vi "libdaq_adc_read_analog.vi"(0 "error in (no error)":errorcluster, 1 "device_name":string, 2 "module_name":string, 4 "datalen_ch":u32, 5 "channel_list":u8[](array[numeric])=[1]) -> (14 "error out":errorcluster, 15 "device_name":string, 16 "module_name":string, 18 "databuf":dbl[][](array[numeric]))   [LabVIEW 2010, in "libdaqVI.lvlib"]
doc: "读取ADC模块的采样电压值。该函数内部已经完成了从ADC编码到实际电压值的转换操作过程，对用户屏蔽了ADC的位数，模拟通道的放大倍数等参数，简化了ADC模块的使用过程"
uses:
  libdaqVI.lvlib
  dll/daqlib.dll
panel:
  out "actuallen":u32
  out "databuf":dbl[](array[numeric])
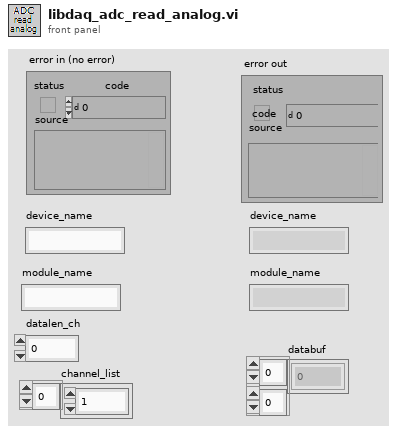
[diagram p1: front panel]
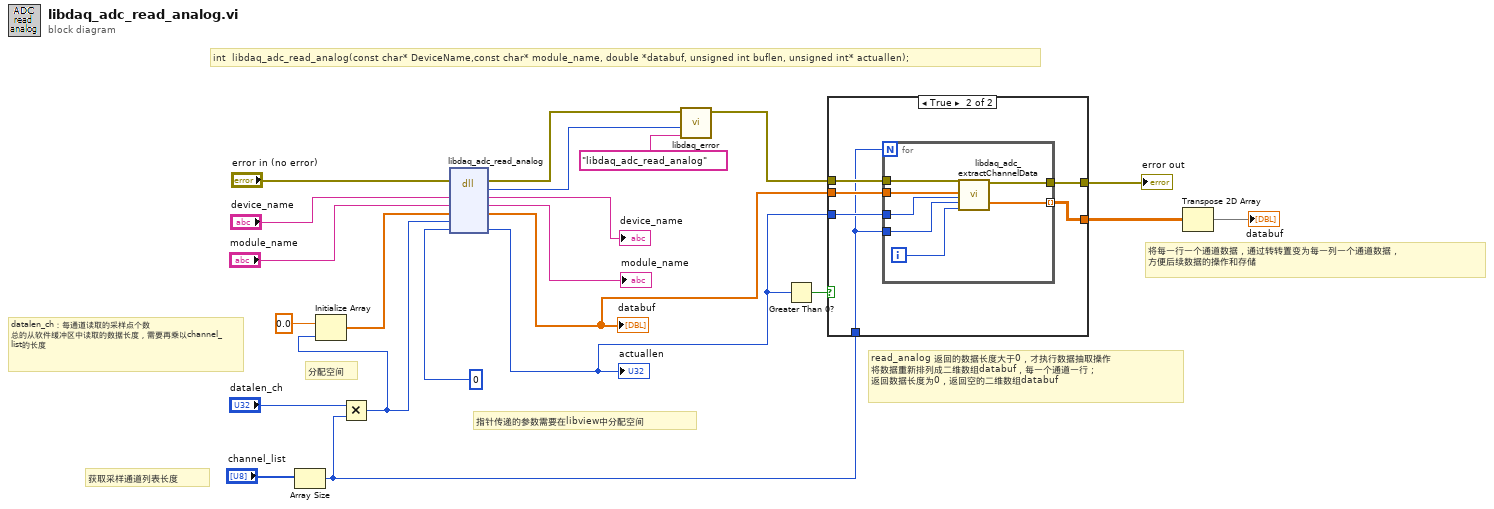
[diagram p0: block diagram]
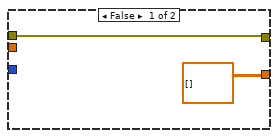
[diagram p2: hidden frame]
diagram:
  # "分配空间"
  # "datalen_ch：每通道读取的采样点个数\n总的从软件缓冲区中读取的数据长度，需要再乘以channel_list的长度"
  # "将每一行一个通道数据，通过转转置变为每一列一个通道数据，\n方便后续数据的操作和存储"
  # "read_analog 返回的数据长度大于0，才执行数据抽取操作\n将数据重新排列成二维数组databuf，每一个通道一行；\n返回数据长度为0，返回空的二维数组databuf"
  # "获取采样通道列表长度"
  # "指针传递的参数需要在libview中分配空间"
  # "int  libdaq_adc_read_analog(const char* DeviceName,const char* module_name, double *databuf, unsigned int buflen, unsigned int* actuallen);"
  n1 = Array Size(array="channel_list") -> (size(s)=w1:i32)
  n2 = Multiply(x="datalen_ch", y=w1) -> (x*y=w2:u32)
  n3 = Initialize Array(0.0, w2) -> (w18:dbl[])
  n4 = dll-call lib="E:/Product/Example/DAQ-USB3212/Labview/labview_2010/libdaqVI/dll/daqlib.dll" fn="libdaq_adc_read_analog"(error in="error in (no error)", "device_name"="device_name", "module_name"="module_name", "databuf"=w18, "buflen"=w2, "actuallen"=u32 0 ("actuallen 2")) -> (error out=w12:errorcluster, "return type"=w10:i32, "device_name"=→"device_name":string, "module_name"=→"module_name":string, "databuf"=w13:dbl[], "actuallen"=w7:u32)  [unwired: 3 in, 1 out]
  "databuf" <- w13
  "actuallen" <- w7
  n5 = call "libdaq_error.vi"("error source"="libdaq_adc_read_analog", "error code"=w10, "错误输入（无错误）"=w12) -> ("错误输出"=w11:errorcluster)  [unwired: 8 in]
  n6 = Greater Than 0?(x=w7) -> (x > 0?=w6:bool)
  n7 = case shown="True" w6 {
    tunnel: [w24 w30] -> w14
    tunnel: w13 -> [_ w29]
    tunnel: w7 -> [_ w28]
    tunnel: w11 -> [w24 w27]
    tunnel: w1 -> [_ w26]
    tunnel: [dbl[][] [] ("ch_databuf") w25] -> w8
    frame False {
    }
    frame True {
      n8 = for {
        N: w26 -> [_]
        tunnel: w29 -> [w36]
        tunnel: w28 -> [w35]
        tunnel: w26 -> [w34]
        tunnel: w27 -> [w33]
        tunnel: [w37] -> w30
        tunnel: [w31] -> w25 mode=indexing
        i -> [w32]
        n9 = call "libdaq_adc_extractChannelData.vi"("error in (no error)"=w33, "all_databuf"=w36, "all_buflen"=w35, "ch_listlen"=w34, "ch_index"=w32) -> ("error out"=w37:errorcluster, "ch_databuf"=w31:dbl[])  [unwired: 13 in]
      }
    }
  }
  "error out" <- w14
  n10 = Transpose 2D Array(2D array=w8) -> (transposed array=→"databuf":dbl[][])
